vi "_OLS_Main.vi"() -> ()   [LabVIEW 2024]
uses:
  Control Definitions/Def Results2.ctl
  Control Definitions/Def TestState.ctl
  Control Definitions/Global 1.vi
  Control Definitions/Global 2.vi
panel:
  in  "SimPV":bool
  out "TEST State Out":T1=enum."Filling"
  out "Ctl Sig":dbl=100.0
  out "Ch B  Sim":dbl
  out "Ch A  Sim":dbl
  out "Root Path":path=path "C:/Users/ff107/OneDrive/Documents/GitHub/PWC-OLS"
  out "File Name":string
  out "Time(ms)":dbl=221.000000000016
  in  "Tank Cal Table":T2={"LSe"=8.5, "LKe"=4.0782, "LMe"=5.542, "LKf"=7.004, "LMf"=2.619, "LSf"=2.0}
  in  "State Msg":enum16{"INIT", "IDLE", "STOP", "FILL", "DRAIN"}(ring)=enum."STOP"
  out "Level":bool=TRUE
  out "DataQ":bool=TRUE
  in  "ChA":dbl(slide)=24.489795918367346 scale=0.0..1200.0
  in  "ChB":dbl(slide)=36.73469387755102 scale=0.0..1200.0
  in  "ChB +100":bool
  in  "ChA +100":bool
  in  "Check":bool
  out "Laser (raw)":dbl=5.418700218200684
  out "Results out":T3=[[{"Fill"=0.0, "Drain"=0.0, "Status"=1, "Resistor"=100.77651728439153}, {"Fill"=0.0, "Drain"=0.0, "Status"=1, "Resistor"=100.51009270770467}], [{"Fill"=7.4414529208790405, "Drain"=0.0, "Status"=10, "Resistor"=199.9225077433029}, {"Fill"=7.238431105656106, "Drain"=0.0, "Status"=5, "Resistor"=199.90723695805426}], [{"Fill"=7.01332844493592, "Drain"=0.0, "Status"=5, "Resistor"=299.5771992355265}, {"Fill"=6.753456462357763, "Drain"=0.0, "Status"=10, "Resistor"=299.405945542382}], [{"Fill"=6.5453388658426634, "Drain"=0.0, "Status"=10, "Resistor"=398.9472825404134}, {"Fill"=6.2984555038112795, "Drain"=0.0, "Status"=10, "Resistor"=398.8781708461997}], [{"Fill"=6.077648954516121, "Drain"=0.0, "Status"=10, "Resistor"=498.9171881446158}, {"Fill"=5.838658669949018, "Drain"=0.0, "Status"=10, "Resistor"=498.9668209325864}], [{"Fill"=5.635836474430779, "Drain"=0.0, "Status"=10, "Resistor"=599.1164295543886}, {"Fill"=5.372367525813369, "Drain"=0.0, "Status"=10, "Resistor"=599.0753796448585}], [{"Fill"=5.159054576363429, "Drain"=0.0, "Status"=10, "Resistor"=699.4116005363627}, {"Fill"=4.928457133151359, "Drain"=0.0, "Status"=10, "Resistor"=699.1833846499306}], [{"Fill"=4.711946933490899, "Drain"=0.0, "Status"=10, "Resistor"=799.7085090018842}, {"Fill"=4.472056930994641, "Drain"=0.0, "Status"=10, "Resistor"=799.8411539311372}], [{"Fill"=0.0, "Drain"=0.0, "Status"=2, "Resistor"=0.0}, {"Fill"=0.0, "Drain"=0.0, "Status"=0, "Resistor"=0.0}], [{"Fill"=0.0, "Drain"=0.0, "Status"=0, "Resistor"=0.0}, {"Fill"=0.0, "Drain"=0.0, "Status"=0, "Resistor"=0.0}], [{"Fill"=0.0, "Drain"=0.0, "Status"=0, "Resistor"=0.0}, {"Fill"=0.0, "Drain"=0.0, "Status"=0, "Resistor"=0.0}]] {"Resistor" format="%.1f"; "Drain" format="%.3f"; "Fill" format="%.3f"}
  in  "DUT":i16=1
  in  "Pump JOG":bool
  in  "Run Test":bool=TRUE
  in  "Normal":cluster{u32, u32}[](array[cluster])=[{16711680, 1244948}]
  in  "Sim Color":cluster{u32, u32}[](array[cluster])=[{16774656, 1244948}]
  out "Level \nStatus":bool=TRUE
  out "DataQ\nStatus":bool=TRUE
  in  "Level SP":dbl(slide)=2.6 scale=8.5..2.0
  in  "Level PV":dbl(slide)=4.203692297209104 scale=8.5..2.0
  in  "Flow Rate %":dbl(knob)=100.0 scale=0.0..100.0
  out "Level":dbl=4.203692297209104 format="%.3f"
  in  "Drain":bool
  in  "Fill":bool
  in  "Simulate":bool
  out "TEST NME":string="OLR001--Junk"
  out "DataQ Input":T4(graph)={"ChA Ohms"=799.7643554010987, "ChB Ohms"=799.7713366200159, "Laser (raw)"=5.343100070953369}
  out "Time Stamp":timestamp=timestamp(3801643928.5713105 s since 1904-01-01)
  in  "stop":bool
  out "ChB Ohms":dbl=799.966848563534 format="%.1f"
  out "ChA Ohms":dbl=899.5202427178965 format="%.1f"
  # "Calibration & Scaling Table\n               Tank         Key          Ref\n               Scale        Level        Measure\n\n\n\nEmpty\n\n\nFull"
  # "8.5   1.7752   7.844\n\n2.0   6.112    3.511"
  # "CHA"
  # "CHB"
  # "Resistance   Fill        Drain"
  # "Resistance   Fill        Drain"
  # "Simulated Instrument Inputs"
  # "PUMP"
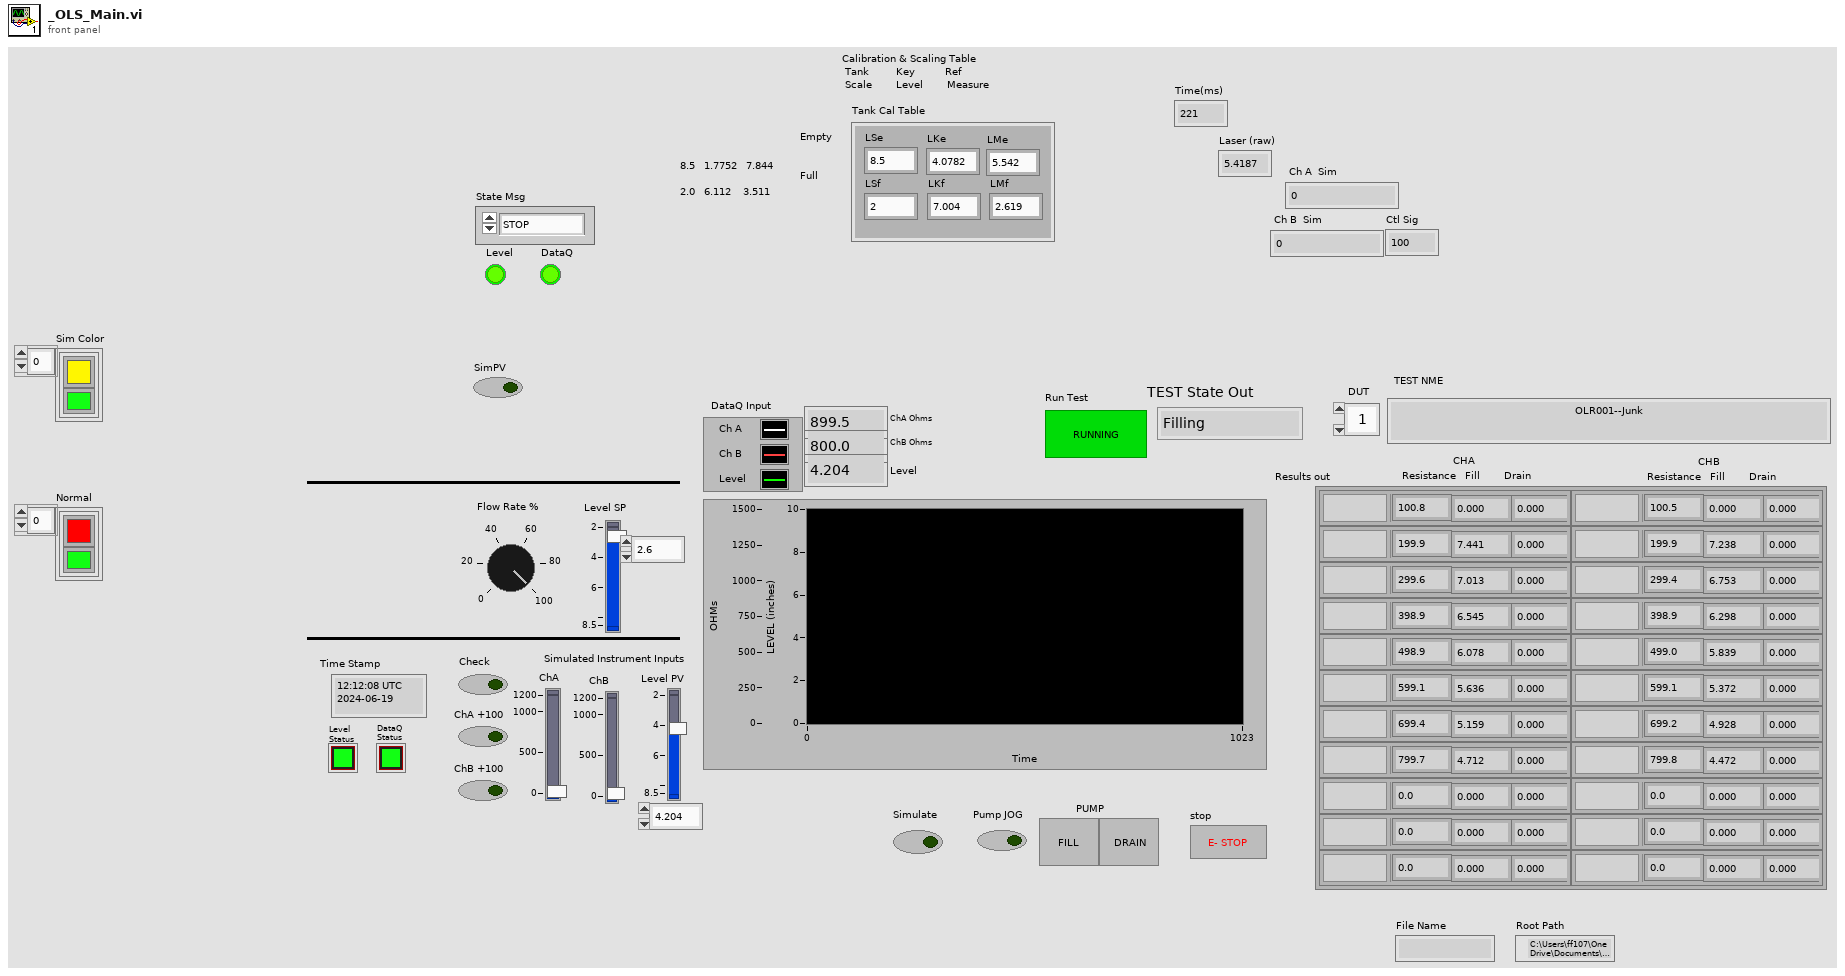
[diagram p1: front panel]
types:
  T1 = typedef "Def TestState.ctl" = enum16{"MANUAL", "Start", "Pre-Fill", "Pre-Drain", "Start-Record", "Filling", "FULL", "Draining", "EMPTY", "Done"}
  T2 = cluster{"LSe":dbl, "LKe":dbl, "LMe":dbl, "LKf":dbl, "LMf":dbl, "LSf":dbl}
  T3 = typedef "Def Results2.ctl" = cluster{"Fill":dbl, "Drain":dbl, "Status":i16, "Resistor":dbl}[][]
  T4 = cluster{"ChA Ohms":dbl, "ChB Ohms":dbl, "Laser (raw)":dbl}
  T5 = cluster{"Level \nStatus":refnum<vi>, "DataQ\nStatus":refnum<vi>}
  T6 = typedef "Def PumpCtlRefs.ctl" = cluster{"Fill ":refnum<vi>, "Drain":refnum<vi>, "Level PV":refnum<vi>, "Flow Rate%":refnum<vi>, "Run Test":refnum<vi>, "Sim":refnum<vi>, "Jog":refnum<vi>, "Level SP":refnum<vi>}
  T7 = typedef "Def FullCfg.ctl" = cluster{"Bench Config":T8, "Test Value Table ":dbl[][], "Table Col Titles":string[][], "Pump CtlRef In":T6, "Bench Status":T9}
  T8 = typedef "Def BenchCfg.ctl" = cluster{"Name":string, cluster{"Step Levels":dbl, "Tolerance":dbl, "Sample Rate":dbl, "Resistor":dbl, "M Level Cal":dbl, "[B Level Cal":dbl, "Max Fill Rate":dbl, "Empty Inches":dbl, "Full Inches":dbl}}
  T9 = typedef "Def Bench Status.ctl" = cluster{"Pump Status":refnum<vi>, "Instrumnet\n Status":refnum<vi>}
  T10 = typedef "Def CalCoef.ctl" = cluster{"M":dbl, "B":dbl, "Mc":dbl, "Bc":dbl, "LMe":dbl}
  T11 = enum16{"MANUAL", "Start", "Filling", "FULL", "Draining", "EMPTY", "Done"}
  T12 = cluster{"Resistor":dbl, "Fill":dbl, "Drain":dbl, "Status":i16}
  T13 = cluster{"Resistor":dbl, "Fill":dbl, "Drain":dbl, "Status":i16}[][]
  T14 = cluster{"Ch A   Ohms":dbl, " Ch B  Ohms":dbl, "Level OUt":dbl}
  T15 = typedef "Ded Spec RNG.ctl" = cluster{"Specs":dbl[], "Index(n)":i32, "LUT Status":T16, "Index(n-1)":i32}
  T16 = typedef "Ded LUT_Status.ctl" = cluster{"ChA/!ChB":bool, "Drain/!Fill":bool, "In Range?":bool, "Switch Range?":bool, "Measure R?":bool, "Vaild R?":bool}
  T17 = typedef "Def Measure.ctl" = cluster{"ChA R":dbl, "ChB R":dbl, "Level PV":dbl}
  T18 = cluster{"Resistor":dbl, "Fill":dbl, "Drain":dbl, "Resistor":dbl}[][]
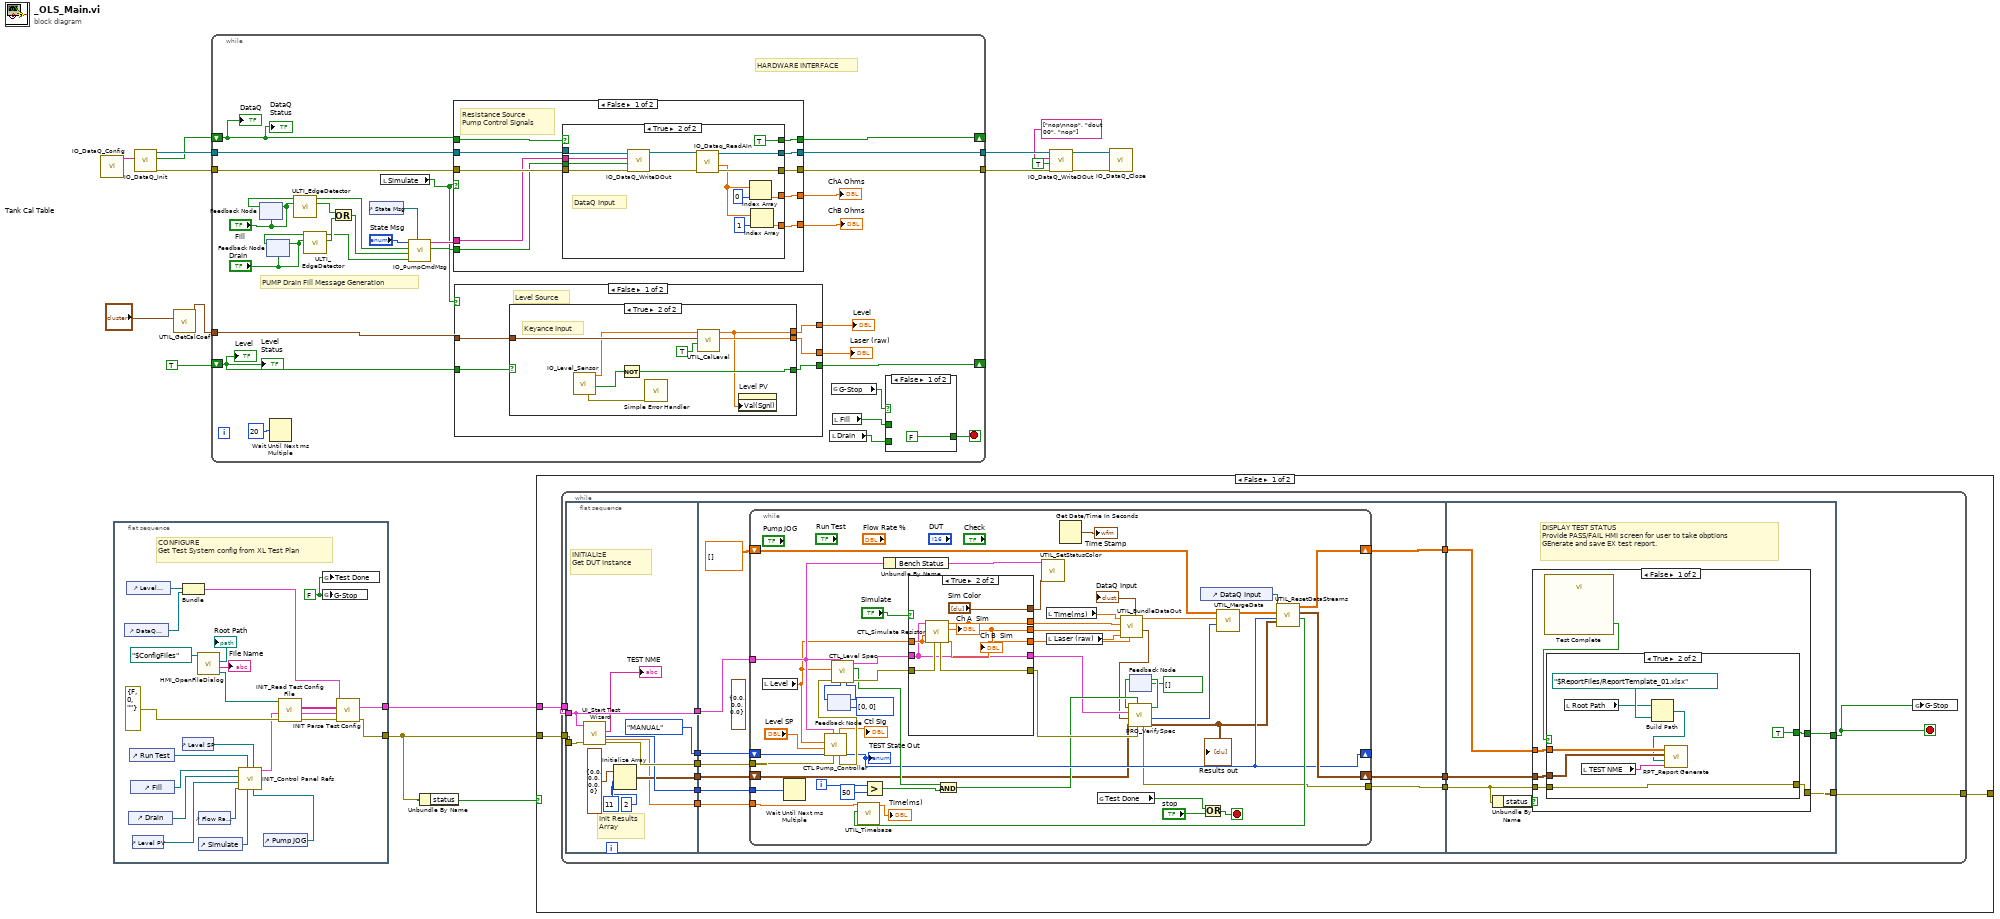
[diagram p0: block diagram]
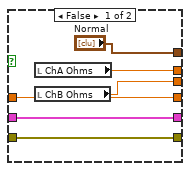
[diagram p2: hidden frame]
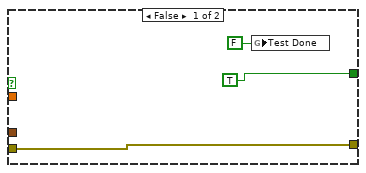
[diagram p3: hidden frame]
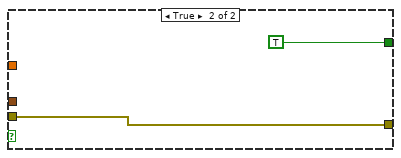
[diagram p4: hidden frame]
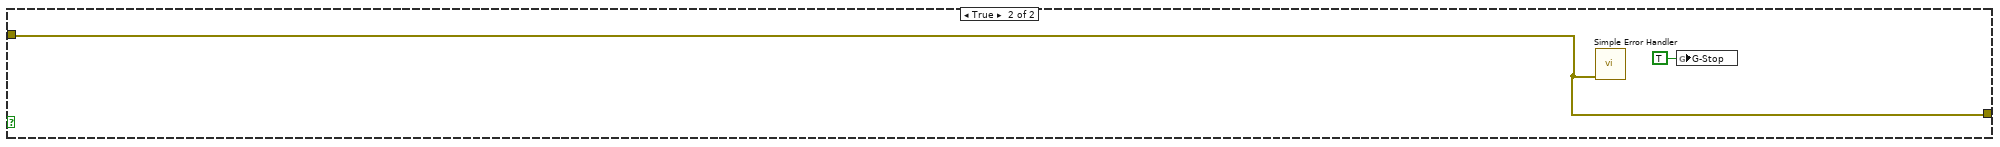
[diagram p5: hidden frame]
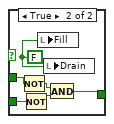
[diagram p6: hidden frame]
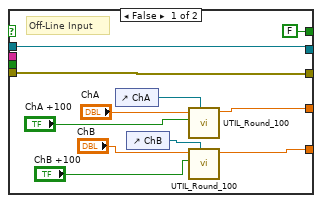
[diagram p7: hidden frame]
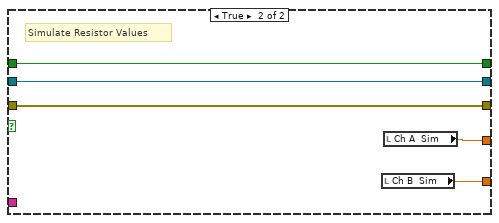
[diagram p8: hidden frame]
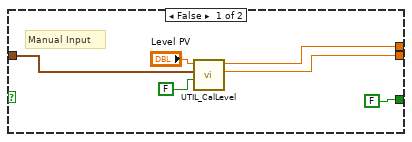
[diagram p9: hidden frame]
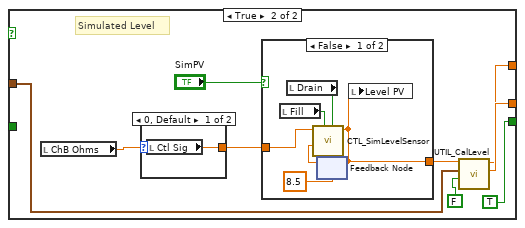
[diagram p10: hidden frame]
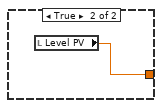
[diagram p11: hidden frame]
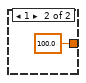
[diagram p12: hidden frame]
diagram:
  n1 = call "IO_DataQ_Config.vi"() -> ("Init Message"=w16:string[])  [unwired: 11 in]
  n2 = flat-sequence {
    tunnel: [w36] -> w7
    tunnel: [w26] -> w10
    frame #0 {
      w21 = FALSE ("G-Stop")
      # "CONFIGURE\nGet Test System config from XL Test Plan"
      n3 = control-ref of="DataQ\nStatus"() -> (w23:refnum<vi>)
      n4 = control-ref of="Level \nStatus"() -> (w35:refnum<vi>)
      n5 = control-ref of="Drain"() -> (w37:refnum<vi>)
      n6 = control-ref of="Run Test"() -> (w28:refnum<vi>)
      n7 = control-ref of="Fill"() -> (w29:refnum<vi>)
      n8 = control-ref of="Level PV"() -> (w32:refnum<vi>)
      n9 = Bundle("Level \nStatus"=w35, "DataQ\nStatus"=w23) -> (w33:T5)  [unwired: 1 in]
      n10 = control-ref of="Level SP"() -> (w22:refnum<vi>)
      n11 = call "HMI_OpenFileDialog.vi"("relative path"=path "$ConfigFiles") -> ("selected path"=w17:path, "File Name"=→"File Name":string, "Root Path"=→"Root Path":path)  [unwired: 8 in]
      n12 = control-ref of="Flow Rate %"() -> (w30:refnum<vi>)
      n13 = control-ref of="Simulate"() -> (w25:refnum<vi>)
      n14 = control-ref of="Pump JOG"() -> (w24:refnum<vi>)
      n15 = call "INIT_Control Panel Refs.vi"("Jog"=w24, "Level SP"=w22, "Sim"=w25, "Run Test"=w28, "Flow Rate %"=w30, "Level PV"=w32, "Drain"=w37, "Fill"=w29) -> ("PumpCtlRef out"=w34:T6)  [unwired: 3 in]
      n16 = call "INIT_Read Test Config File.vi"("error in (no error)"=errorcluster {"status"=FALSE, "code"=0, "source"=""}, "Path"=w17) -> ("error out 2"=w27:errorcluster, "Config\nFile Data"=w31:string[][])  [unwired: 8 in]
      n17 = global write "Global 1.vi" "G-Stop"(w21) -> ()
      n18 = global write "Global 2.vi" "Test Done"(w21) -> ()
      n19 = call "INIT Parse Test Config.vi"("error in (no error)"=w27, "Pump CtlRef In"=w34, "All XL Input"=w31, "Bench Status"=w33) -> ("error out"=w36:errorcluster, "Full Config"=w26:T7)  [unwired: 6 in]
    }
  }
  n20 = call "IO_DataQ_Init.vi"("Command\nList"=w16) -> ("error out"=w14:errorcluster, "Connected?"=w13:bool, "VISA resource name out"=w15:refnum<visa-resource-name>)  [unwired: 8 in]
  n21 = call "UTIL_GetCalCoef.vi"("Cal Table"="Tank Cal Table") -> ("Cal Coef out"=w11:T10)  [unwired: 10 in]
  n22 = while {
    shift-right: [w65] -> _
    shift-left: TRUE ("Pump \nStatus") -> [w45]
    tunnel: w15 -> [w64]
    tunnel: w14 -> [w63]
    tunnel: [w61] -> w6
    tunnel: [w62] -> w4
    shift-right: [w60] -> _
    shift-left: w13 -> [w48]
    tunnel: w11 -> [w44]
    stop <- w41 stop-if-true
    # "PUMP Drain Fill Message Generation"
    # "HARDWARE INTERFACE"
    n23 = feedback #1("Fill") -> (w58:bool)
    n24 = feedback-in #1("Fill") -> ()
    n25 = feedback #2("Drain") -> (w59:bool)
    n26 = feedback-in #2("Drain") -> ()
    n27 = Wait Until Next ms Multiple(millisecond multiple=u32 20) -> ()  [unwired: 1 out]
    n28 = call "ULTI_EdgeDetector.vi"("IN (N)"="Fill", "IN (N+2)"=w58) -> ("Neg Edge"=w56:bool, "Pos Edge"=w55:bool)  [unwired: 8 in]
    n29 = call "ULTI_EdgeDetector.vi"("IN (N)"="Drain", "IN (N+2)"=w59) -> ("Neg Edge"=w54:bool, "Pos Edge"=w53:bool)  [unwired: 8 in]
    n30 = Or(x=w56, y=w54) -> (x .or. y?=w57:bool)
    n31 = control-ref of="State Msg"() -> (w51:refnum<vi>)
    n32 = local read "Simulate"() -> (w43:bool)
    n33 = call "IO_PumpCmdMsg.vi"("State Ref"=w51, "Drain Signal"=w53, "Stop Signal"=w57, "FIll Signal"=w55, "State\n in"="State Msg") -> ("Msg Active"=w46:bool, "Message"=w47:string[])  [unwired: 5 in]
    n34 = case shown="False" w43 {
      tunnel: [w87 w114] -> w69
      tunnel: [w86 w113] -> w68
      tunnel: w64 -> [w78 w116]
      tunnel: w63 -> [w81 w115]
      tunnel: [w85 w115] -> w62
      tunnel: [w84 w116] -> w61
      tunnel: [w83 w117] -> w60
      tunnel: w48 -> [w82 w117]
      tunnel: w47 -> [w79 _]
      tunnel: w46 -> [w80 _]
      frame False {
        # "Resistance Source\nPump Control Signals"
        n35 = case shown="True" w82 {
          tunnel: [w91 w106] -> w87
          tunnel: [w92 w107] -> w86
          tunnel: [w93 w112] -> w84
          tunnel: [w94 w111] -> w85
          tunnel: [FALSE TRUE] -> w83
          tunnel: w81 -> [w94 w104]
          tunnel: w80 -> [_ w103]
          tunnel: w79 -> [_ w102]
          tunnel: w78 -> [w93 w101]
          frame False {
            # "Off-Line Input"
            n36 = control-ref of="ChA"() -> (w90:refnum<vi>)
            n37 = control-ref of="ChB"() -> (w88:refnum<vi>)
            n38 = call "UTIL_Round_100.vi"("Num Refnum"=w90, "100"="ChA +100", "IN"="ChA") -> ("OUT"=w92:dbl)  [unwired: 8 in]
            n39 = call "UTIL_Round_100.vi"("Num Refnum"=w88, "100"="ChB +100", "IN"="ChB") -> ("OUT"=w91:dbl)  [unwired: 8 in]
          }
          frame True {
            # "DataQ Input"
            n40 = call "IO_DataQ_WriteDOut.vi"("error in (no error)"=w104, "Msg Active"=w103, "Message"=w102, "VISA Refnum in"=w101) -> ("error out"=w100:errorcluster, "VISA Refnum out"=w99:refnum<visa-resource-name>)  [unwired: 5 in, 1 out]
            n41 = call "IO_Dataq_ReadAIn.vi"("error in (no error)"=w100, "VISA Refnum in"=w99) -> ("error out"=w111:errorcluster, "Outputs"=w108:dbl[], "VISA Refnum out"=w112:refnum<visa-resource-name>)  [unwired: 5 in, 2 out]
            n42 = Index Array(array=w108, index=0) -> (element=w107:dbl)
            n43 = Index Array(array=w108, index=1) -> (element=w106:dbl)
          }
        }
      }
      frame True {
        # "Simulate Resistor Values"
        n44 = local read "Ch B  Sim"() -> (w114:dbl)
        n45 = local read "Ch A  Sim"() -> (w113:dbl)
      }
    }
    "ChA Ohms" <- w68
    "ChB Ohms" <- w69
    n46 = case shown="False" w43 {
      tunnel: [w122 w141] -> w67
      tunnel: [w121 w144] -> w66
      tunnel: [w118 TRUE] -> w65
      tunnel: w45 -> [w120 _]
      tunnel: w44 -> [w119 w142]
      frame False {
        # "Level Source"
        n47 = case shown="True" w120 {
          tunnel: [w126 w129] -> w122
          tunnel: [w125 w134] -> w121
          tunnel: [FALSE ("status") w133] -> w118
          tunnel: w119 -> [w127 w135]
          frame False {
            # "Manual Input"
            n48 = call "UTIL_CalLevel.vi"("Key is In?"=FALSE, "Cal Coef in"=w127, "Input"="Level PV") -> ("PVc"=w125:dbl, "PVs"=w126:dbl)  [unwired: 7 in]
          }
          frame True {
            # "Keyance Input"
            n49 = call "IO_Level_Sensor.vi"() -> ("status"=w131:bool, "PV (raw)"=w132:dbl, "error OUT"=w130:errorcluster)  [unwired: 9 in]
            n50 = Not(x=w131) -> (.not. x?=w133:bool)
            n51 = call <vilib>:"Simple Error Handler.vi"("error in (no error)"=w130) -> ()  [unwired: 4 in, 5 out]
            n52 = call "UTIL_CalLevel.vi"("Key is In?"=TRUE, "Cal Coef in"=w135, "Input"=w132) -> ("PVc"=w134:dbl, "PVs"=w129:dbl)  [unwired: 7 in]
            n53 = property on="Level PV" class="Slide (strict)"("Val(Sgnl)"=w129) -> ()  [unwired: 2 in, 2 out]
          }
        }
      }
      frame True {
        # "Simulated Level"
        n54 = local read "ChB Ohms"() -> (w139:dbl)
        n55 = case shown="0, Default" w139 {
          tunnel: [w153 100.0 ("Ctl Sig")] -> w140
          frame 0, Default {
            n56 = local read "Ctl Sig"() -> (w153:dbl)
          }
          frame 1 {
          }
        }
        n57 = case shown="False" "SimPV" {
          tunnel: w140 -> [w150 _]
          tunnel: [w146 w152] -> w138
          frame False {
            n58 = local read "Fill"() -> (w151:bool)
            n59 = local read "Drain"() -> (w147:bool)
            n60 = feedback #3(8.5 ("PV Level Inch")) -> (w148:dbl)
            n61 = call "CTL_SimLevelSensor.vi"("Drain IN"=w147, "Fill IN"=w151, "Level PV in"=w148, "Flow Rate %"=w150) -> ("PV Level Inch"=w146:dbl)  [unwired: 7 in]
            n62 = feedback-in #3(w146) -> ()
            n63 = local write "Level PV"(w146) -> ()
          }
          frame True {
            n64 = local read "Level PV"() -> (w152:dbl)
          }
        }
        n65 = call "UTIL_CalLevel.vi"("Key is In?"=FALSE, "Cal Coef in"=w142, "Input"=w138) -> ("PVc"=w144:dbl, "PVs"=w141:dbl)  [unwired: 7 in]
      }
    }
    "Level" <- w67
    "Laser (raw)" <- w66
    n66 = local read "Drain"() -> (w39:bool)
    n67 = global read "Global 1.vi" "G-Stop"() -> (w42:bool)
    n68 = local read "Fill"() -> (w40:bool)
    n69 = case shown="False" w42 {
      tunnel: [FALSE w73] -> w41
      tunnel: w40 -> [_ w75]
      tunnel: w39 -> [_ w72]
      frame False {
      }
      frame True {
        w77 = FALSE
        n70 = Not(x=w75) -> (.not. x?=w76:bool)
        n71 = Not(x=w72) -> (.not. x?=w74:bool)
        n72 = local write "Fill"(w77) -> ()
        n73 = local write "Drain"(w77) -> ()
        n74 = And(x=w76, y=w74) -> (x .and. y?=w73:bool)
      }
    }
    "DataQ\nStatus" <- w48
    "Level \nStatus" <- w45
    "DataQ" <- w48
    "Level" <- w45
  }
  n75 = Unbundle By Name(w7) -> ("status"=w9:bool)
  n76 = case shown="False" w9 {
    tunnel: w7 -> [w157 w281]
    tunnel: w10 -> [w156 _]
    tunnel: [w155 w281] -> _
    frame False {
      n77 = while {
        tunnel: w157 -> [w167]
        tunnel: w156 -> [w165]
        tunnel: [w160] -> w155
        stop <- w159 stop-if-true
        n78 = flat-sequence {
          tunnel: [w179] -> w169
          tunnel: [w180] -> w168
          tunnel: w167 -> [w181]
          tunnel: [w178] -> w166
          tunnel: w165 -> [w178]
          tunnel: [T11."MANUAL" ("TEST STATUS Out")] -> w164
          tunnel: [w173] -> w163
          tunnel: [w172] -> w158
          tunnel: [w184] -> w170
          tunnel: w169 -> [w190]
          tunnel: w168 -> [w191]
          tunnel: w166 -> [w189]
          tunnel: w164 -> [w182]
          tunnel: w163 -> [w188]
          tunnel: [w187] -> w162
          tunnel: [w186] -> w161
          tunnel: w158 -> [w185]
          tunnel: w170 -> [w261]
          tunnel: [w260] -> w159
          tunnel: [w258] -> w160
          tunnel: w162 -> [w257]
          tunnel: w161 -> [w256]
          frame #0 {
            # "Init Results\nArray"
            # "INITIALIzE\nGet DUT Instance"
            n79 = call "UI_Start Test Wizard.vi"("error in (no error)"=w181, "Full Config"=w178) -> ("error out"=w180:errorcluster, "Time Base mS"=w179:i32, "Title"=→"TEST NME":string, "Sample Rate"=w172:dbl)  [unwired: 4 in]
            n80 = Initialize Array(T12 {"Resistor"=0.0, "Fill"=0.0, "Drain"=0.0, "Status"=0} ("Cluster 2"), 11 ("dimension size"), 2 ("dimension size")) -> (w173:T13)
          }
          frame #1 {
            (unwired) T14 {"Ch A   Ohms"=0.0, " Ch B  Ohms"=0.0, "Level OUt"=0.0}
            n81 = while {
              tunnel: w190 -> [w240]
              tunnel: w191 -> [w221]
              tunnel: [w205] -> w184
              tunnel: w189 -> [w227]
              shift-right: [w212] -> w186
              shift-left: w188 -> [w204]
              tunnel: w185 -> [w218]
              shift-right: [w214] -> w187
              shift-left: dbl[][] [] ("Array") -> [w195]
              shift-right: [w209] -> _
              shift-left: w182 -> [w208]
              i -> [w217]
              stop <- w237 stop-if-true
              n82 = local read "Level"() -> (w223:dbl)
              n83 = Wait Until Next ms Multiple(millisecond multiple=w240) -> ()  [unwired: 1 out]
              n84 = call "CTL Pump_Controller.vi"("error in (no error)"=w221, "Full Config"=w227, "TEST State In"=w208, "Level SP"="Level SP", "Level PV"=w223) -> ("TEST State Out"=w209:T1, "error out"=w220:errorcluster, "Ctl Sig"=→"Ctl Sig":dbl)  [unwired: 2 in, 2 out]
              "TEST State Out" <- w209
              n85 = feedback #4(i32[] [0, 0] ("Index(n-1) In")) -> (w230:i32[])
              n86 = call "CTL_Level Spec.vi"("Index(n-1) In"=w230, "Full Config"=w227, "error in (no error)"=w220, "Level IN inches"=w223) -> ("error out"=w226:errorcluster, "Enable"=w219:bool, "aSpec Out"=w225:T15[], "Index(n-1) Out"=w231:i32[])  [unwired: 4 in]
              n87 = feedback-in #4(w231) -> ()
              n88 = Greater?(x=w217, y=50) -> (0:w215:bool)
              n89 = Unbundle By Name(w227) -> ("Bench Status"=w238:T9)
              n90 = case shown="True" "Simulate" {
                tunnel: w226 -> [w248 w251]
                tunnel: [w248 w254] -> w207
                tunnel: ["Normal" "Sim Color"] -> w239
                tunnel: [w246 w253] -> w229
                tunnel: [w245 w252] -> w228
                tunnel: w225 -> [w243 w249]
                tunnel: w223 -> [w244 w250]
                tunnel: [w244 w250] -> w224
                tunnel: [w243 w249] -> w203
                frame False {
                  n91 = local read "ChA Ohms"() -> (w246:dbl)
                  n92 = local read "ChB Ohms"() -> (w245:dbl)
                }
                frame True {
                  n93 = call "CTL_Simulate Resistor.vi"("error in (no error)"=w251, "Level IN"=w250, "aSpec IN"=w249) -> ("Ch B  Ohms"=w252:dbl, "Ch A  Ohms"=w253:dbl, "error out"=w254:errorcluster)  [unwired: 6 in]
                  "Ch A  Sim" <- w253
                  "Ch B  Sim" <- w252
                }
              }
              n94 = And(x=w219, y=w215) -> (x .and. y?=w206:bool)
              n95 = call "UTIL_SetStatusColor.vi"("Colors [4] in"=w239, "Bench Status"=w238) -> ()  [unwired: 10 in]
              n96 = local read "Time(ms)"() -> (w234:dbl)
              n97 = local read "Laser (raw)"() -> (w233:dbl)
              n98 = Get Date/Time In Seconds() -> (seconds since 1Jan1904=→"Time Stamp":timestamp)
              n99 = global read "Global 2.vi" "Test Done"() -> (w235:bool)
              n100 = call "UTIL_BundleDataOut.vi"("Level PV"=w224, "Laser (raw)"=w233, "ChB Ohms"=w228, "ChA Ohms"=w229, "Time (ms)"=w234) -> ("Measure"=w202:T17, "Data Out"=w197:dbl[], "Chart Data"=→"DataQ Input":T4)  [unwired: 3 in, 1 out]
              n101 = feedback #5(bool[] [] ("Switched Out")) -> (w199:bool[])
              n102 = call "PRO_VerifySpec.vi"("error in (no error)"=w207, "Enable"=w206, "Results in"=w204, "Measure In"=w202, "aSpec In"=w203, "Switched In"=w199) -> ("Results out"=w201:T3, "Status Code"=w196:i32, "Switched Out"=w200:bool[], "error out"=w205:errorcluster)  [unwired: 2 in]
              "Results out" <- w201
              n103 = feedback-in #5(w200) -> ()
              n104 = control-ref of="DataQ Input"() -> (w192:refnum<vi>)
              n105 = Or(x=w235, y="stop") -> (x .or. y?=w237:bool)
              n106 = call "UTIL_MergeData.vi"("Status Code"=w196, "New Data"=w197, "Data In"=w195) -> ("Data out"=w194:dbl[][])  [unwired: 8 in]
              n107 = call "UTIL_ResetDataStreams.vi"("Results in"=w201, "TEST State Out"=w209, "Data in"=w194, "WaveformChart in"=w192) -> ("Value (Signaling)"=w210:bool, "Results out 2"=w212:T18, "Array"=w214:dbl[][])  [unwired: 5 in]
              n108 = call "UTIL_Timebase.vi"("Reset"=w210, "Sample Rate"=w218) -> ("Time(ms)"=→"Time(ms)":dbl)  [unwired: 9 in]
            }
          }
          frame #2 {
            # "DISPLAY TEST STATUS\nProvide PASS/FAIL HMI screen for user to take obptions\nGEnerate and save EX test report."
            n109 = Unbundle By Name(w261) -> ("status"=w259:bool)
            n110 = case shown="False" w259 {
              tunnel: w261 -> [w265 w279]
              tunnel: [w266 TRUE] -> w260
              tunnel: [w264 w279] -> w258
              tunnel: w257 -> [w263 _]
              tunnel: w256 -> [w262 _]
              frame False {
                n111 = call "Test Complete"() -> ("SAVE"=w267:bool)  [unwired: 18 in, 1 out]
                n112 = case shown="True" w267 {
                  tunnel: [TRUE TRUE] -> w266
                  tunnel: w265 -> [w269 w277]
                  tunnel: [w269 w277] -> w264
                  tunnel: w263 -> [_ w276]
                  tunnel: w262 -> [_ w275]
                  frame False {
                    n113 = global write "Global 2.vi" "Test Done"(FALSE ("Test Done")) -> ()
                  }
                  frame True {
                    n114 = local read "Root Path"() -> (w273:path)
                    n115 = local read "TEST NME"() -> (w271:string)
                    n116 = Build Path(base path=w273, name or relative path=path "$ReportFiles/ReportTemplate_01.xlsx") -> (appended path=w272:path)
                    n117 = call "RPT_Report Generate.vi"("Report Name"=w271, "template"=w272, "Results"=w275, "Wave Data"=w276) -> ()  [unwired: 8 in]
                  }
                }
              }
              frame True {
              }
            }
          }
        }
        n118 = global write "Global 1.vi" "G-Stop"(w159) -> ()
      }
    }
    frame True {
      n119 = call <vilib>:"Simple Error Handler.vi"("error in (no error)"=w281) -> ()  [unwired: 4 in, 5 out]
      n120 = global write "Global 1.vi" "G-Stop"(TRUE ("G-Stop")) -> ()
    }
  }
  n121 = call "IO_DataQ_WriteDOut.vi"("error in (no error)"=w4, "Msg Active"=TRUE, "Message"=string[] ["nop\nnop", "dout 00", "nop"], "VISA Refnum in"=w6) -> ("error out"=w3:errorcluster, "VISA Refnum out"=w5:refnum<visa-resource-name>)  [unwired: 5 in, 1 out]
  n122 = call "IO_DataQ_Close.vi"("error in"=w3, "VISA resource name"=w5) -> ()  [unwired: 9 in, 1 out]
